vi "read image.vi"(8 "error in (no error)":errorcluster, 11 "CCDCamera in":refnum<class "Simulated Camera.lvclass">) -> (0 "error out":errorcluster, 2 "Image Graph":u16[][](array[numeric]), 3 "CCDCamera out":refnum<class "Simulated Camera.lvclass">)   [LabVIEW 2018, in "Simulated Camera.lvclass"]
uses:
  Simulated Camera.lvclass
  Simulated Camera.lvclass/Simulated Camera.ctl
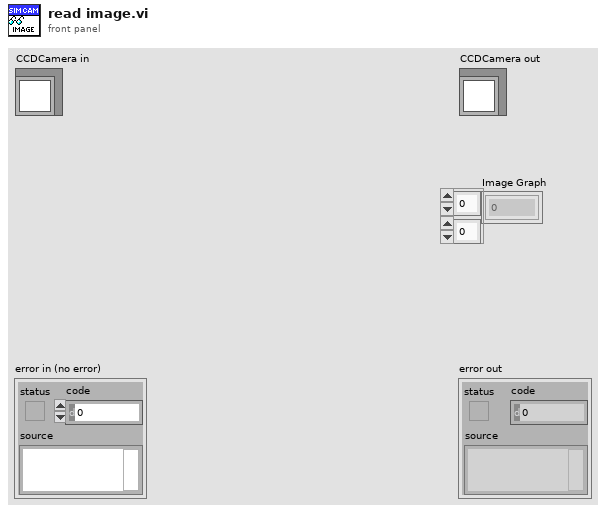
[diagram p1: front panel]
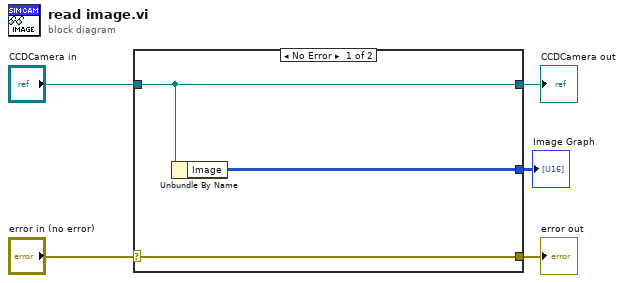
[diagram p0: block diagram]
diagram:
  n1 = case shown="No Error" "error in (no error)" {
    selector: "error in (no error)" -> [w8 w9]
    tunnel: [w8 w9] -> w4
    tunnel: [w7 w10] -> w2
    tunnel: "CCDCamera in" -> [w7 w10]
    tunnel: [w6 _] -> w1
    frame No Error {
      n2 = Unbundle By Name(w7) -> ("Image"=w6:u16[][])
    }
    frame Error {
    }
  }
  "error out" <- w4
  "CCDCamera out" <- w2
  "Image Graph" <- w1
